vi "BLE_Verify_Connect.vi"(0 ".NET Refnum in":refnum<k24>, 5 "ConnectBLE":refnum<k24>, 11 "error in (no error)":errorcluster) -> (4 ".NET Refnum out":refnum<k24>, 6 "ConnectBLE":refnum<k24>, 8 "IsCompleted":bool, 10 "Status":i32(ring) items=["Created", "WaitingForActivation", "WaitingToRun", "Running", "WaitingForChildrenToComplete", "RanToCompletion", "Canceled", "Faulted"], 14 "Result":string, 15 "error out":errorcluster)   [LabVIEW 2019]
uses:
  C:/Users/chrismadlax/Desktop/LabVIEW-BLE-Driver/BLELib.dll
  BLELib.dll
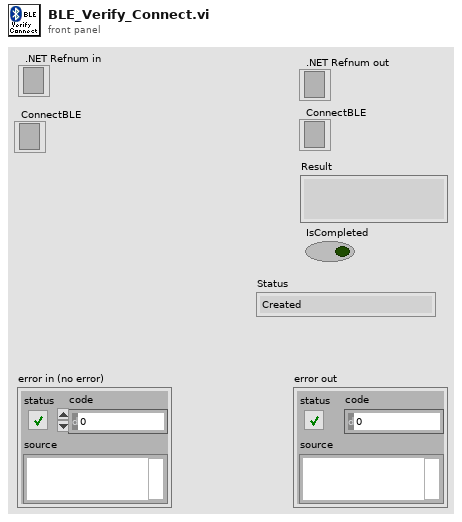
[diagram p1: front panel]
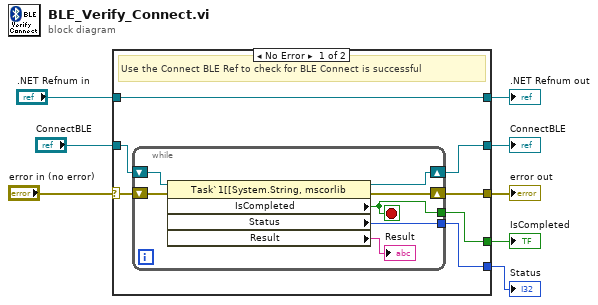
[diagram p0: block diagram]
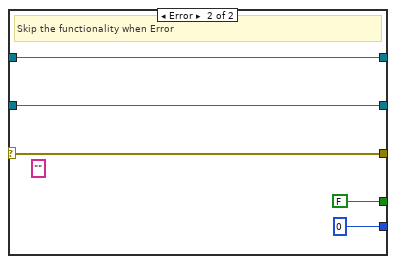
[diagram p2: hidden frame]
diagram:
  n1 = case shown="No Error" "error in (no error)" {
    selector: "error in (no error)" -> [w14 w27]
    tunnel: [w15 w27] -> w8
    tunnel: [w10 FALSE ("IsCompleted")] -> w6
    tunnel: "ConnectBLE" -> [w13 w26]
    tunnel: [w9 0 ("Status")] -> w5
    tunnel: [w12 w26] -> w1
    tunnel: [w11 w23] -> w4
    tunnel: ".NET Refnum in" -> [w11 w23]
    frame No Error {
      # "Use the Connect BLE Ref to check for BLE Connect is successful"
      n2 = while {
        shift-right: [w20] -> w15
        shift-left: w14 -> [w19]
        shift-right: [w16] -> w12
        shift-left: w13 -> [w22]
        tunnel: [w21] -> w10
        tunnel: [w18] -> w9
        stop <- w21 stop-if-true
        n3 = property class="Task`1[[System.String, mscorlib"(reference=w22, error in=w19) -> (reference out=w16:refnum<k24>, error out=w20:errorcluster, "IsCompleted"=w21:bool, "Status"=w18:i32, "Result"=→"Result":string)
      }
    }
    frame Error {
      (unwired) "" ("Result")
      # "Skip the functionality when Error"
    }
  }
  "error out" <- w8
  "IsCompleted" <- w6
  "Status" <- w5
  "ConnectBLE" <- w1
  ".NET Refnum out" <- w4
